vi "ControlPointUnderMouse.vi"(0 "FSM.Edge In":refnum<class "FSM.Edge.lvclass">, 9 "Coords":T1) -> (4 "FSM.Edge Out":refnum<class "FSM.Edge.lvclass">, 8 "control point?":bool, 10 "controlIndex":i32)   [LabVIEW 2020, in "FSM.Edge.lvclass"]
uses:
  FSM.Edge.lvclass
  <vilib>/Utility/miscctls.llb/LVPoint32TypeDef.ctl
  FSM.Edge.lvclass/FSM.Edge.ctl
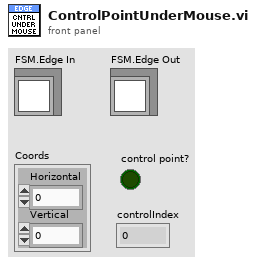
[diagram p1: front panel]
types:
  T1 = typedef "LVPoint32TypeDef.ctl" = cluster{"Horizontal":i32, "Vertical":i32}
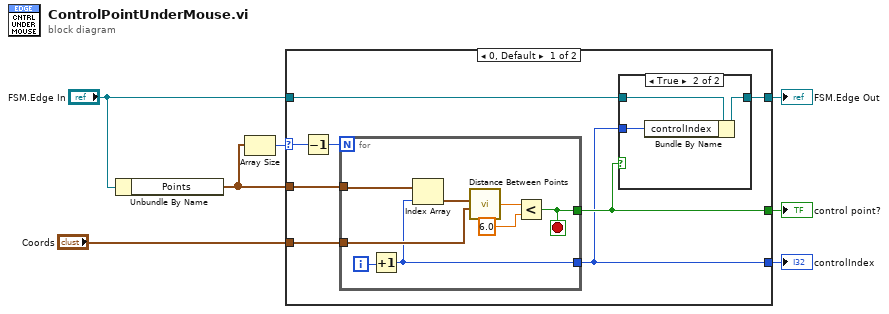
[diagram p0: block diagram]
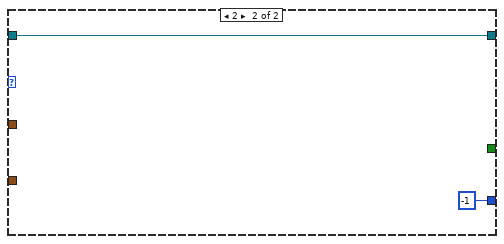
[diagram p3: hidden frame]
diagram:
  n1 = Unbundle By Name("FSM.Edge In") -> ("Points"=w4:cluster{"x":i16, "y":i16}[])
  n2 = Array Size(array=w4) -> (size(s)=w5:i32)
  n3 = case shown="0, Default" w5 {
    selector: w5 -> [w14 _]
    tunnel: "Coords" -> [w15 _]
    tunnel: [w11 _] -> w6
    tunnel: w4 -> [w13 _]
    tunnel: [w8 -1] -> w3
    tunnel: "FSM.Edge In" -> [w10 w28]
    tunnel: [w9 w28] -> w1
    frame 0, Default {
      n4 = Decrement(x=w14) -> (x-1=w12:i32)
      n5 = for {
        N: w12 -> [_]
        tunnel: w13 -> [w23]
        tunnel: w15 -> [w27]
        tunnel: [w24] -> w11
        tunnel: [w20] -> w8
        i -> [w21]
        stop <- w24 stop-if-true
        n6 = Increment(x=w21) -> (x+1=w20:i32)
        n7 = Index Array(array=w23, index=w20) -> (element=w22:cluster{"x":i16, "y":i16})
        n8 = call "Distance Between Points.vi"("B"=w27, "A"=w22) -> ("distance"=w26:dbl)  [unwired: 4 in]
        n9 = Less?(x=w26, y=6.0) -> (x < y?=w24:bool)
      }
      n10 = case shown="True" w11 {
        tunnel: w10 -> [w16 w19]
        tunnel: [w16 w18] -> w9
        tunnel: w8 -> [_ w17]
        frame False {
        }
        frame True {
          n11 = Bundle By Name(cluster=w19, "controlIndex"=w17) -> (w18:refnum<class "FSM.Edge.lvclass">)
        }
      }
    }
    frame 2 {
    }
  }
  "FSM.Edge Out" <- w1
  "control point?" <- w6
  "controlIndex" <- w3
